vi "Detail_Fixture 1_8.vi"() -> ()   [LabVIEW 2017]
uses:
  <vilib>/Platform/TimedLoop/XDataNode/timing_clust.ctl
  <vilib>/Platform/TimedLoop/XDataNode/nitl_modes.ctl
  <vilib>/Platform/TimedLoop/XDataNode/wakeup.ctl
  <vilib>/platform/TimedLoop/XDataNode/XDataNode.xnode
  <vilib>/Platform/TimedLoop/XDataNode/XDNodeRunTimeDep.lvlib
panel:
  out "FIXTURE No.":string
  out "Vision Pad":string
  out "Vision Pin":string
  out "QR Code":string
  out "LIN WDW Lock":string
  out "LIN DR Up":string
  out "LIN DR Down":string
  out "LIN DR Auto":string
  out "LIN AS Up":string
  out "LIN AS Down":string
  out "LIN AS Auto":string
  out "RL Man Up":string
  out "RL Man Down":string
  out "FL Auto Up":string
  out "FL Auto Down":string
  out "FL Man Down":string
  out "FL Man Up":string
  out "RR Man Down":string
  out "RR Man Up":string
  out "FR Auto Down":string
  out "FR Auto Up":string
  out "FR Man Down":string
  out "FR Man Up":string
  out "Door Unlocked":string
  out "Door Lock":string
  out "WDW Unlocked":string
  out "WDW Locked":string
  out "Megga Test":string
  out "RESULT":string
  out "LASER  No.":string
  out "LANE  No.":string
  out "PRODUCT No.":string
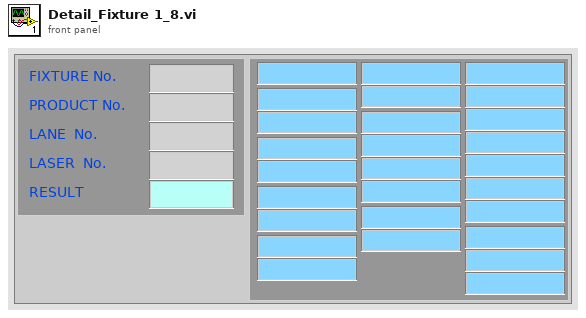
[diagram p1: front panel]
types:
  T1 = typedef "XDNodeRunTimeDep.lvlib/timing_clust.ctl" = cluster{"Expected End [f-1]":u64, "Actual End [f-1]":u64, "Finished Late? [f-1]":bool, "Expected End [i-1]":u64, "Actual End [i-1]":u64, "Finished Late? [i-1]":bool, "Expected Start [i]":u64, "Actual Start [i]":u64, "Expected Start [f]":u64, "Actual Start [f]":u64, "Source Name":string, "Structure Name":string, "Period":i64, "Deadline":i64, "Offset":i64, "Start":i64, "Priority":i32, "Timeout":i32, "Mode":T2, "Wakeup Reason":T3, "Error":errorcluster, "Source Type":string, "Secondary Source Type":string, "Global End Time":u64, "Global Start Time":u64, "Frame Duration":u64, "Iteration Duration":u64, "Assigned CPU":i32, "I/O Scan Engine Mode":u32}
  T2 = typedef "XDNodeRunTimeDep.lvlib/nitl_modes.ctl" = enum32{"No Change", "Process missed periods, maintain original phase", "Discard missed periods, maintain original phase", "Process missed periods, ignore original phase", "Discard missed periods, ignore original phase"}
  T3 = typedef "XDNodeRunTimeDep.lvlib/wakeup.ctl" = enum32{"Normal", "Aborted", "Asynchronous wakeup", "Timing source error", "Timed loop error", "Timeout"}
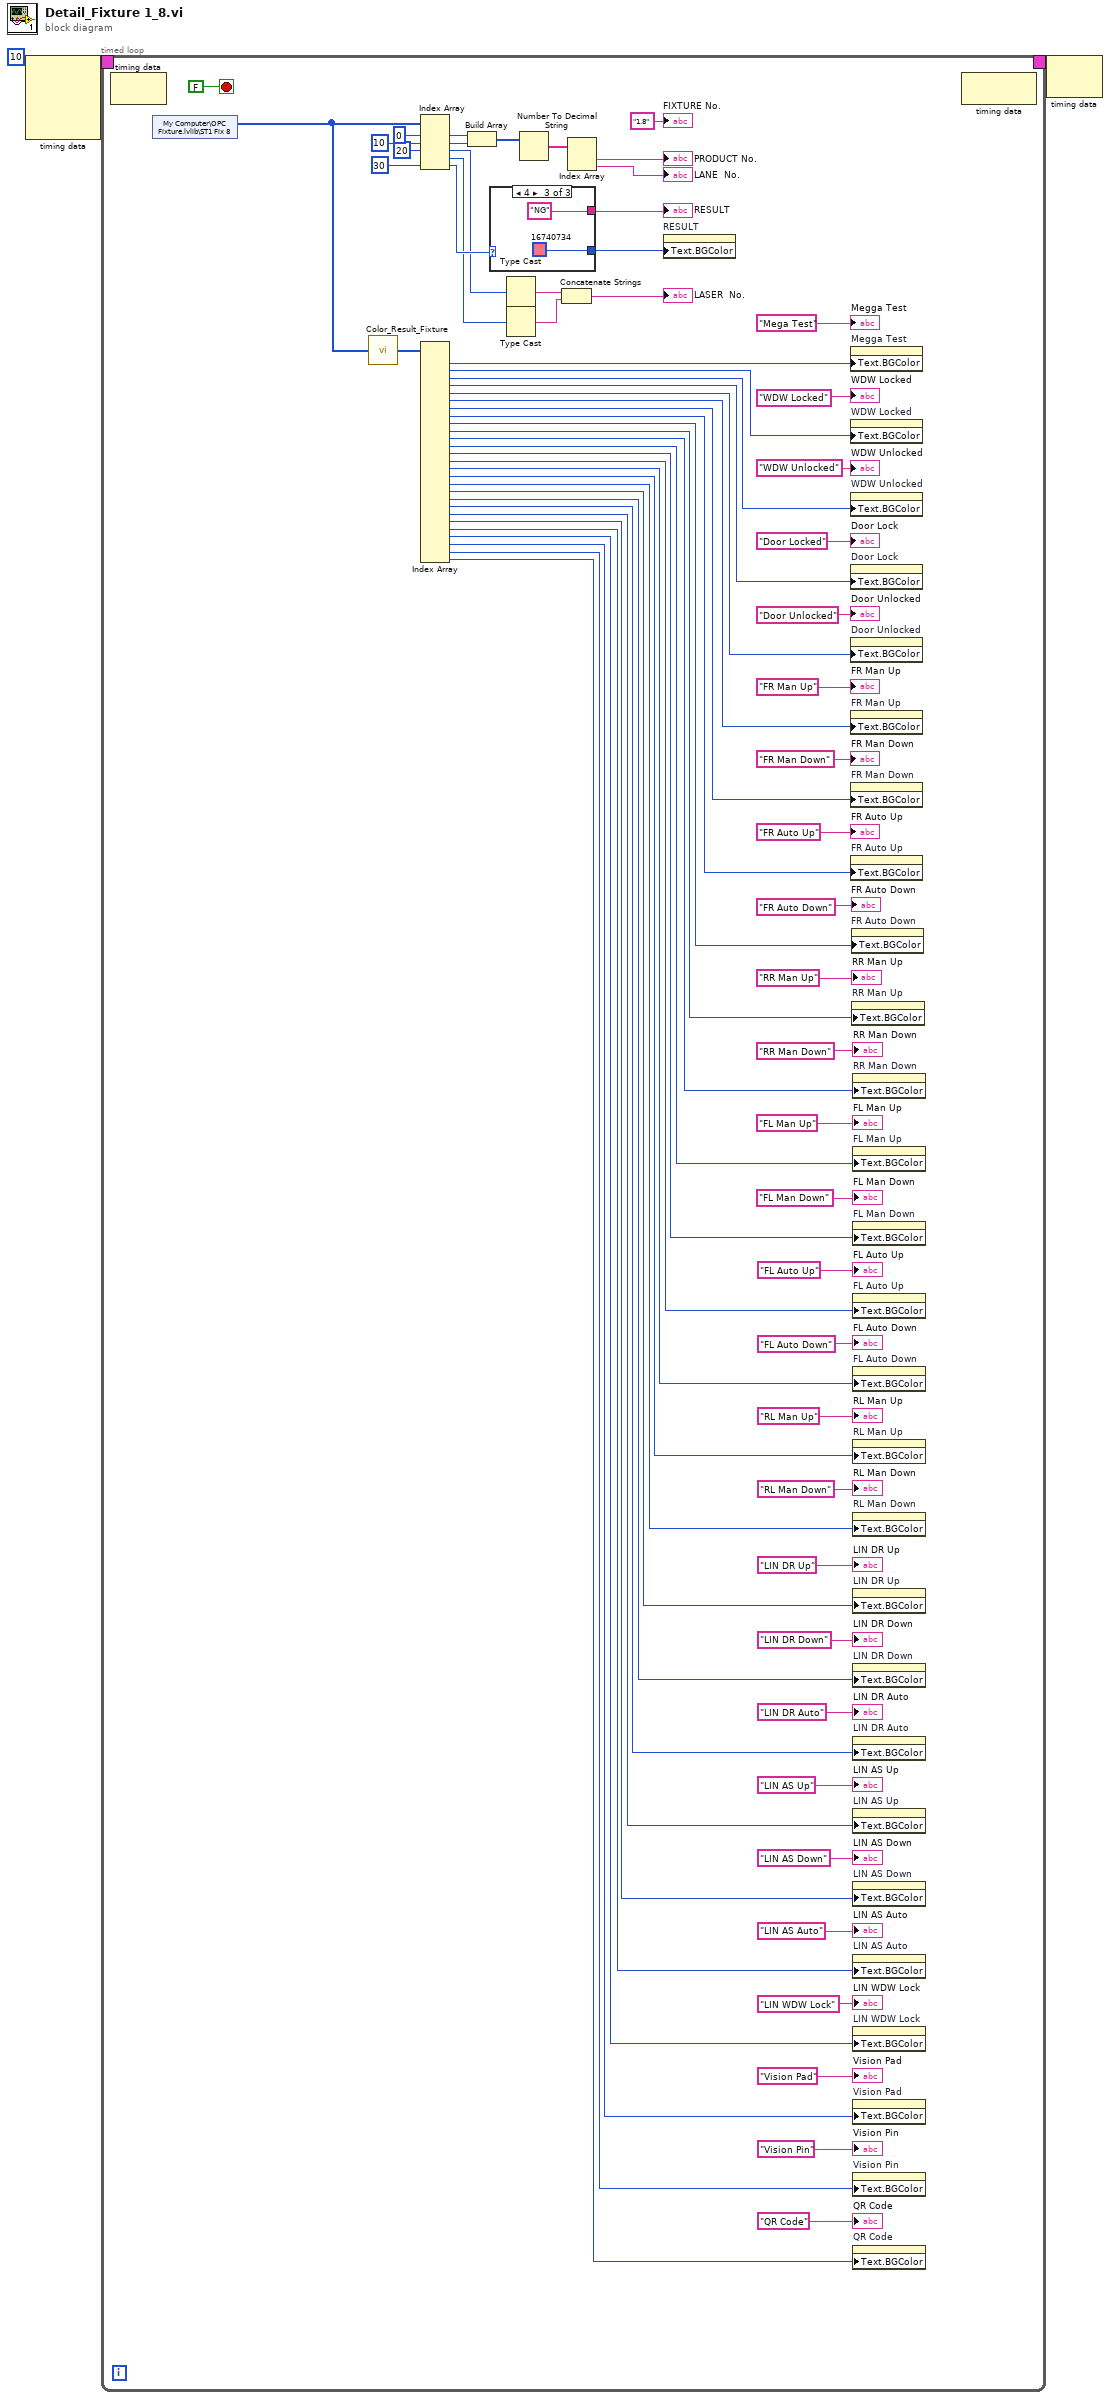
[diagram p0: block diagram]
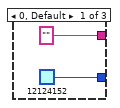
[diagram p2: hidden frame]
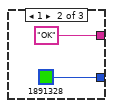
[diagram p3: hidden frame]
diagram:
  n1 = node-c288(i64 10 ("Period")) -> (w3:T1)  [unwired: 3 in]
  n2 = timed-loop {
    timing: w3 -> [_]
    timing-out: [_] -> w2
    stop <- FALSE stop-if-true
    n3 = node-c288() -> ()  [unwired: 1 in, 1 out]
    n4 = shared-variable "My Computer\\OPC Fixture.lvlib\\ST1 Fix 8"() -> (w79:u16[])  [unwired: 1 in, 1 out]
    n5 = call "Color_Result_Fixture.vi"("Fixture_Data"=w79) -> ("Array_Color_Result"=w75:u32[])  [unwired: 4 in]
    n6 = Index Array(array=w79, index #1=0 ("index"), index #2=10 ("index"), index #3=20 ("index"), index #5=30 ("index")) -> (element #1=w74:u16, element #2=w73:u16, element #3=w4:u16, element #4=w5:u16, element #5=w6:u16)  [unwired: 1 in]
    n7 = Index Array(array=w75) -> (element #1=w64:u32, element #2=w62:u32, element #3=w60:u32, element #4=w58:u32, element #5=w56:u32, element #6=w54:u32, element #7=w52:u32, element #8=w50:u32, element #9=w48:u32, element #10=w46:u32, element #11=w44:u32, element #12=w42:u32, element #13=w40:u32, element #14=w37:u32, element #15=w36:u32, element #16=w33:u32, element #17=w32:u32, element #18=w21:u32, element #19=w20:u32, element #20=w19:u32, element #21=w18:u32, element #22=w17:u32, element #23=w16:u32, element #24=w15:u32, element #25=w14:u32, element #26=w13:u32, element #27=w12:u32)  [unwired: 27 in]
    n8 = Build Array(w74, w73) -> (w72:u16[])
    n9 = case shown="4" w6 {
      tunnel: [u32 12124152 u32 1891328 u32 16740734] -> w67
      tunnel: ["" "OK" "NG"] -> w66
      frame 0, Default {
      }
      frame 1 {
      }
      frame 4 {
      }
    }
    "RESULT" <- w66
    n10 = Type Cast(x=w4) -> (*(type *) &x=w10:string)  [unwired: 1 in]
    n11 = Type Cast(x=w5) -> (*(type *) &x=w9:string)  [unwired: 1 in]
    n12 = Number To Decimal String(number=w72) -> (decimal integer string=w71:string[])  [unwired: 1 in]
    n13 = Concatenate Strings(w10, w9) -> (→"LASER  No.":string)
    n14 = Index Array(array=w71) -> (element #1=→"PRODUCT No.":string, element #2=→"LANE  No.":string)  [unwired: 2 in]
    n15 = property on="RESULT" class="Str"("Text.BGColor"=w67) -> ()  [unwired: 2 in, 2 out]
    n16 = property on="Megga Test" class="Str"("Text.BGColor"=w64) -> ()  [unwired: 2 in, 2 out]
    n17 = property on="WDW Locked" class="Str"("Text.BGColor"=w62) -> ()  [unwired: 2 in, 2 out]
    n18 = property on="WDW Unlocked" class="Str"("Text.BGColor"=w60) -> ()  [unwired: 2 in, 2 out]
    n19 = property on="Door Lock" class="Str"("Text.BGColor"=w58) -> ()  [unwired: 2 in, 2 out]
    n20 = property on="Door Unlocked" class="Str"("Text.BGColor"=w56) -> ()  [unwired: 2 in, 2 out]
    n21 = property on="FR Man Up" class="Str"("Text.BGColor"=w54) -> ()  [unwired: 2 in, 2 out]
    n22 = property on="FR Man Down" class="Str"("Text.BGColor"=w52) -> ()  [unwired: 2 in, 2 out]
    n23 = property on="FR Auto Up" class="Str"("Text.BGColor"=w50) -> ()  [unwired: 2 in, 2 out]
    n24 = property on="FR Auto Down" class="Str"("Text.BGColor"=w48) -> ()  [unwired: 2 in, 2 out]
    n25 = property on="RR Man Up" class="Str"("Text.BGColor"=w46) -> ()  [unwired: 2 in, 2 out]
    n26 = property on="RR Man Down" class="Str"("Text.BGColor"=w44) -> ()  [unwired: 2 in, 2 out]
    n27 = property on="FL Man Up" class="Str"("Text.BGColor"=w42) -> ()  [unwired: 2 in, 2 out]
    n28 = property on="FL Man Down" class="Str"("Text.BGColor"=w40) -> ()  [unwired: 2 in, 2 out]
    n29 = property on="FL Auto Up" class="Str"("Text.BGColor"=w37) -> ()  [unwired: 2 in, 2 out]
    n30 = property on="FL Auto Down" class="Str"("Text.BGColor"=w36) -> ()  [unwired: 2 in, 2 out]
    n31 = property on="RL Man Up" class="Str"("Text.BGColor"=w33) -> ()  [unwired: 2 in, 2 out]
    n32 = property on="RL Man Down" class="Str"("Text.BGColor"=w32) -> ()  [unwired: 2 in, 2 out]
    n33 = property on="LIN DR Up" class="Str"("Text.BGColor"=w21) -> ()  [unwired: 2 in, 2 out]
    n34 = property on="LIN DR Down" class="Str"("Text.BGColor"=w20) -> ()  [unwired: 2 in, 2 out]
    n35 = property on="LIN DR Auto" class="Str"("Text.BGColor"=w19) -> ()  [unwired: 2 in, 2 out]
    n36 = property on="LIN AS Up" class="Str"("Text.BGColor"=w18) -> ()  [unwired: 2 in, 2 out]
    n37 = property on="LIN AS Down" class="Str"("Text.BGColor"=w17) -> ()  [unwired: 2 in, 2 out]
    n38 = property on="LIN AS Auto" class="Str"("Text.BGColor"=w16) -> ()  [unwired: 2 in, 2 out]
    n39 = property on="LIN WDW Lock" class="Str"("Text.BGColor"=w15) -> ()  [unwired: 2 in, 2 out]
    n40 = property on="Vision Pad" class="Str"("Text.BGColor"=w14) -> ()  [unwired: 2 in, 2 out]
    n41 = property on="Vision Pin" class="Str"("Text.BGColor"=w13) -> ()  [unwired: 2 in, 2 out]
    n42 = property on="QR Code" class="Str"("Text.BGColor"=w12) -> ()  [unwired: 2 in, 2 out]
    n43 = node-c288() -> ()  [unwired: 1 in, 1 out]
    "Megga Test" <- "Mega Test" ("Megga Test")
    "WDW Locked" <- "WDW Locked" ("Megga Test")
    "WDW Unlocked" <- "WDW Unlocked" ("Megga Test")
    "Door Lock" <- "Door Locked" ("Megga Test")
    "Door Unlocked" <- "Door Unlocked" ("Megga Test")
    "FR Man Up" <- "FR Man Up" ("Megga Test")
    "FR Man Down" <- "FR Man Down" ("Megga Test")
    "FR Auto Up" <- "FR Auto Up" ("Megga Test")
    "FR Auto Down" <- "FR Auto Down" ("Megga Test")
    "RR Man Up" <- "RR Man Up" ("Megga Test")
    "RR Man Down" <- "RR Man Down" ("Megga Test")
    "FL Man Up" <- "FL Man Up" ("Megga Test")
    "FL Man Down" <- "FL Man Down" ("Megga Test")
    "FL Auto Up" <- "FL Auto Up" ("Megga Test")
    "FL Auto Down" <- "FL Auto Down" ("Megga Test")
    "RL Man Up" <- "RL Man Up" ("Megga Test")
    "RL Man Down" <- "RL Man Down" ("Megga Test")
    "LIN DR Up" <- "LIN DR Up" ("Megga Test")
    "LIN DR Down" <- "LIN DR Down" ("Megga Test")
    "LIN DR Auto" <- "LIN DR Auto" ("Megga Test")
    "LIN AS Up" <- "LIN AS Up" ("Megga Test")
    "LIN AS Down" <- "LIN AS Down" ("Megga Test")
    "LIN AS Auto" <- "LIN AS Auto" ("Megga Test")
    "LIN WDW Lock" <- "LIN WDW Lock" ("Megga Test")
    "Vision Pad" <- "Vision Pad" ("Megga Test")
    "Vision Pin" <- "Vision Pin" ("Megga Test")
    "QR Code" <- "QR Code" ("Megga Test")
    "FIXTURE No." <- "1.8" ("FIXTURE No.")
  }
  n44 = node-c288(w2) -> ()  [unwired: 1 out]
